vi "svfa_Window Frequency Response (first derivative, double array).vi"(1 "N (window length)":i32, 2 "window":T1(ring), 3 "f(normalized)":dbl[](array[numeric]) format="%.2f") -> (0 "H'(f)":dbl[](array[numeric]) format="%.2f")   [LabVIEW 2017]
uses:
  <vilib>/addons/_NISVFA/_Spectrum Processing/subVIs/svfa_Window Frequency Response (double).vi
  <vilib>/addons/_NISVFA/_Spectrum Processing/subVIs/svfa_Rect Window Frequency Response.vi
  <vilib>/addons/_NISVFA/_Spectrum Processing/subVIs/svfa_Cosine Window Coefficients.vi
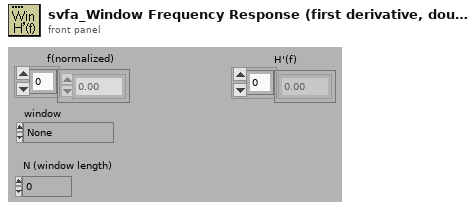
[diagram p1: front panel]
types:
  T1 = enum16{"None ", "Hanning", "Hamming", "Blackman-Harris", "Exact Blackman", "Blackman", "Flat Top", "4 Term B-Harris ", "7 Term B-Harris", "Low Sidelobe"}
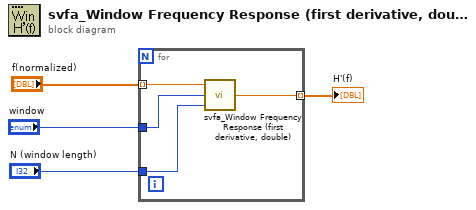
[diagram p0: block diagram]
diagram:
  n1 = for {
    tunnel: "f(normalized)" -> [w8] mode=indexing
    tunnel: "window" -> [w7]
    tunnel: "N (window length)" -> [w6]
    tunnel: [w5] -> w1 mode=indexing
    n2 = call <vilib>:"svfa_Window Frequency Response (first derivative, double).vi"("N (window length)"=w6, "window"=w7, "f(normalized)"=w8) -> ("H'(f)"=w5:dbl)
  }
  "H'(f)" <- w1
